vi "Untitled 2 (SubVI).vi"(6 "Boolean":bool, 7 "Boolean 2":bool, 9 "Boolean 5":bool, 10 "Boolean 6":bool, 11 "Numeric in":i32) -> (1 "Numeric out":i32, 2 "Boolean 3":bool, 3 "Boolean 4":bool)   [LabVIEW 2021]
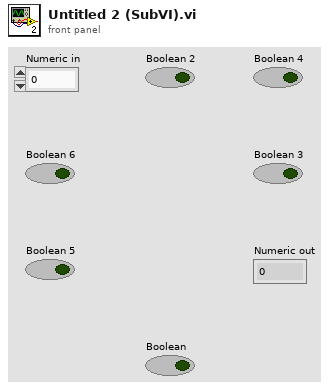
[diagram p1: front panel]
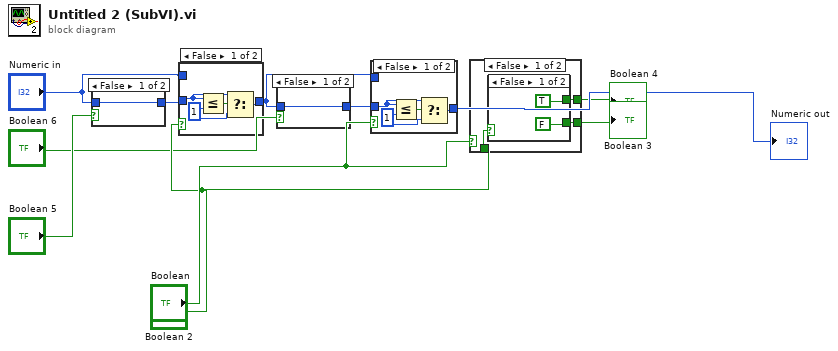
[diagram p0: block diagram]
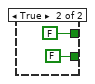
[diagram p2: hidden frame]
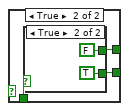
[diagram p3: hidden frame]
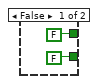
[diagram p4: hidden frame]
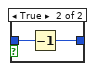
[diagram p6: hidden frame]
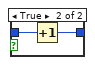
[diagram p8: hidden frame]
diagram:
  n1 = case shown="False" "Boolean 5" {
    tunnel: [w12 w14] -> w3
    tunnel: "Numeric in" -> [w12 w13]
    frame False {
    }
    frame True {
      n2 = Increment(x=w13) -> (x+1=w14:i32)
    }
  }
  n3 = case shown="False" "Boolean 2" {
    tunnel: w3 -> [w17 _]
    tunnel: [w15 w19] -> w5
    tunnel: "Numeric in" -> [_ w19]
    frame False {
      w16 = 1
      n4 = Less Or Equal?(x=w17, y=w16) -> (x <= y?=w18:bool)
      n5 = Select(t=w17, s=w18, f=w16) -> (s? t:f=w15:i32)
    }
    frame True {
    }
  }
  n6 = case shown="False" "Boolean 6" {
    tunnel: w5 -> [w20 w22]
    tunnel: [w20 w21] -> w6
    frame False {
    }
    frame True {
      n7 = Decrement(x=w22) -> (x-1=w21:i32)
    }
  }
  n8 = case shown="False" "Boolean" {
    tunnel: w5 -> [_ w27]
    tunnel: w6 -> [w24 _]
    tunnel: [w23 w27] -> w11
    frame False {
      w25 = 1
      n9 = Less Or Equal?(x=w24, y=w25) -> (x <= y?=w26:bool)
      n10 = Select(t=w24, s=w26, f=w25) -> (s? t:f=w23:i32)
    }
    frame True {
    }
  }
  "Numeric out" <- w11
  n11 = case shown="False" "Boolean" {
    tunnel: "Boolean 2" -> [w28 w37]
    tunnel: [w29 w35] -> w7
    tunnel: [w30 w36] -> w8
    frame False {
      n12 = case shown="False" w28 {
        tunnel: [TRUE FALSE] -> w29
        tunnel: [FALSE FALSE] -> w30
        frame False {
        }
        frame True {
        }
      }
    }
    frame True {
      n13 = case shown="True" w37 {
        tunnel: [FALSE FALSE] -> w35
        tunnel: [FALSE TRUE] -> w36
        frame False {
        }
        frame True {
        }
      }
    }
  }
  "Boolean 3" <- w8
  "Boolean 4" <- w7
